vi "Talker.vi"(0 "Subtract in":refnum<class "Subtract.lvclass">, 5 "Subpanel Ref":refnum<vi>, 11 "Error In":errorcluster) -> (4 "Subtract out":refnum<class "Subtract.lvclass">, 15 "Error Out":errorcluster)   [LabVIEW 2020, in "Subtract.lvclass"]
doc: "Method to call the UI Method. This will pass the object to the UI Method which will do the operation and return the object to the main vi."
uses:
  Subtract.lvclass
  D:/Github Projects/LV_Assignment/Tasks/A18/A18/Classes/Arithmetic_Operations/Arithmetic_Operations.lvclass
  UI.vi
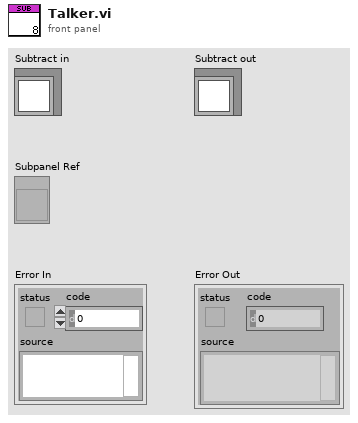
[diagram p1: front panel]
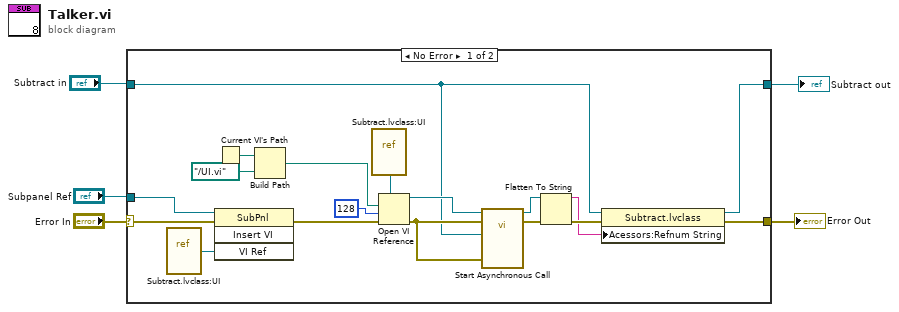
[diagram p0: block diagram]
diagram:
  n1 = case shown="No Error" "Error In" {
    selector: "Error In" -> [w21 w25]
    tunnel: [w11 w25] -> w4
    tunnel: [w10 w24] -> w2
    tunnel: "Subtract in" -> [w9 w24]
    tunnel: "Subpanel Ref" -> [w19 _]
    frame No Error {
      n2 = vi-ref "Subtract.lvclass:UI.vi"() -> (w16:refnum<vi>)
      n3 = invoke on="Invoke Node" class="SubPnl" method="Insert VI"(reference=w19, error in=w21, "VI Ref"=w16) -> (error out=w20:errorcluster)  [unwired: 1 in, 3 out]
      n4 = Current VI's Path() -> (path=w13:path)
      n5 = Build Path(base path=w13, name or relative path=path "../UI.vi") -> (appended path=w12:path)
      n6 = vi-ref "Subtract.lvclass:UI.vi"() -> (w15:refnum<vi>)
      n7 = Open VI Reference(type specifier VI Refnum (for type only)=w15, vi path=w12, options=128, error in (no error)=w20) -> (vi reference=w18:refnum<vi>, error out=w23:errorcluster)  [unwired: 2 in]
      n8 = call-by-ref "Start Asynchronous Call"(reference=w18, error in=w23, "Subtract in"=w9, "Error In"=w23) -> (reference out=w7:refnum<vi>, error out=w17:errorcluster)  [unwired: 11 in, 3 out]
      n9 = Flatten To String(anything=w7, error in (no error)=w17) -> (data string=w6:string, error out=w8:errorcluster)  [unwired: 2 in, 1 out]
      n10 = property class="Subtract.lvclass"(reference=w9, error in=w8, "Acessors:Refnum String"=w6) -> (reference out=w10:refnum<class "Subtract.lvclass">, error out=w11:errorcluster)
    }
    frame Error {
    }
  }
  "Subtract out" <- w2
  "Error Out" <- w4
